vi "AccelerationRetryRoll.vi"(11 "inputInternalData":T5) -> (3 "outputInternalData":T5)   [LabVIEW 2020]
uses:
  Control/AccelerationCurrentRecordIndicator.ctl
  Control/AccelerationBestRecordIndicator.ctl
  CommonControl/Flag.ctl
  Control/AccelerationState.ctl
panel:
  # "Time :"
  # "Entry :"
  # "#1"
  # "#2"
  # "#3"
  # "#4"
  # "Univ. :"
  # "Time :"
  # "Entry :"
  # "#1"
  # "#2"
  # "#3"
  # "#4"
  # "Univ. :"
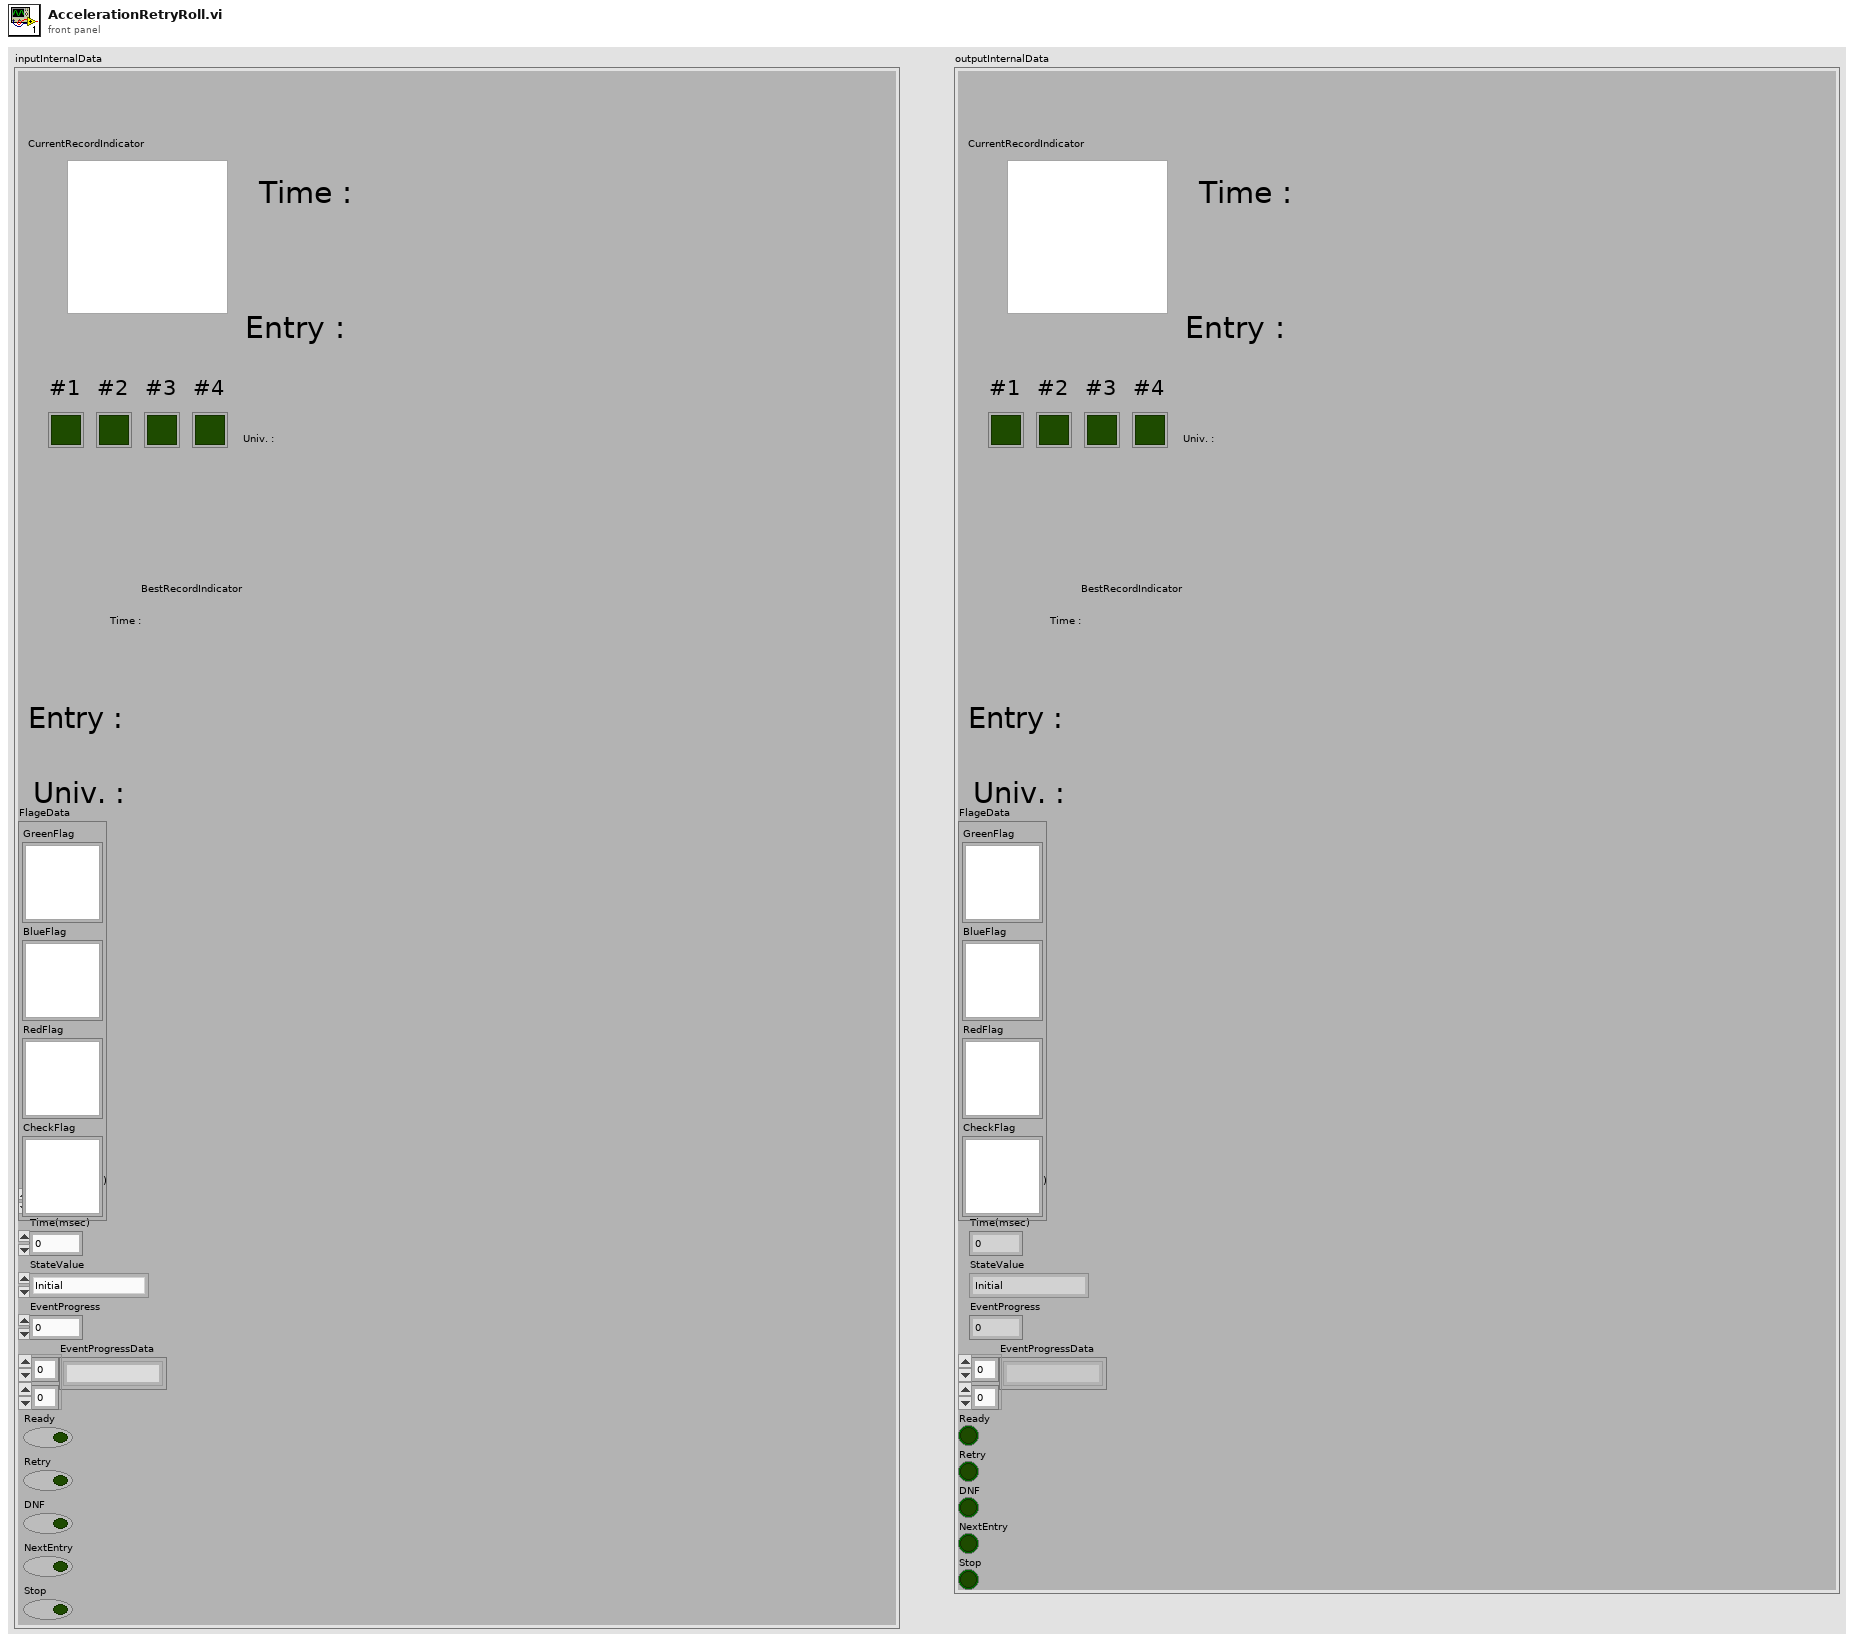
[diagram p1: front panel]
types:
  T1 = typedef "AccelerationCurrentRecordIndicator.ctl" = cluster{"Flag":picture, "Message":string, "Attempt":cluster{"Attempt-1":bool, "Attempt-2":bool, "Attempt-3":bool, "Attempt-4":bool}, "CurrentTime":string, "CurrentEntry":string, "CurrentUniversity":string}
  T2 = typedef "AccelerationBestRecordIndicator.ctl" = cluster{"BestTime":string, "BestEntry":string, "BestUniv":string}
  T3 = typedef "Flag.ctl" = cluster{"GreenFlag":picture, "BlueFlag":picture, "RedFlag":picture, "CheckFlag":picture}
  T4 = typedef "AccelerationState.ctl" = enum16{"Initial", "InputInfomation", "Ready", "Running", "FinshRunning", "LogRecord", "HardwareRelease", "WaittingforNext", "ProgramStop"}
  T5 = cluster{"CurrentRecordIndicator":T1, "BestRecordIndicator":T2, "FlageData":T3, "RefTime(msec)":i64, "Time(msec)":i64, "StateValue":T4, "EventProgress":sgl, "EventProgressData":string[][], "Ready":bool, "Retry":bool, "DNF":bool, "NextEntry":bool, "Stop":bool}
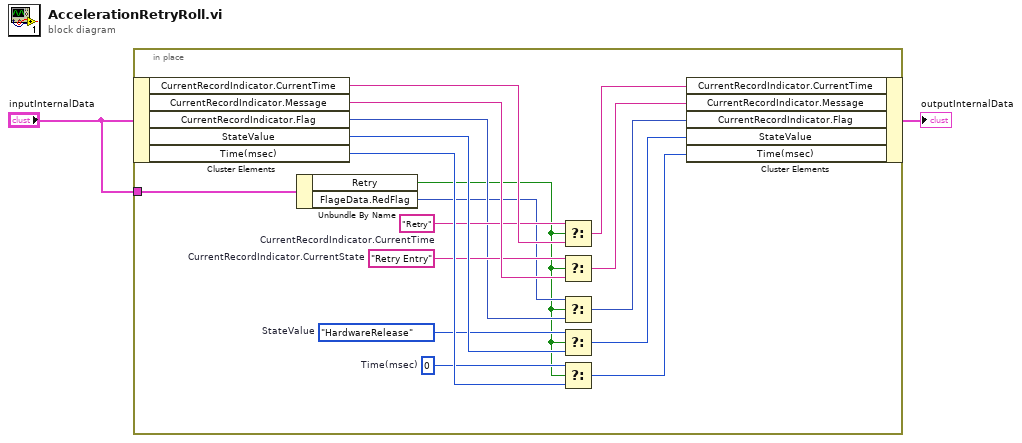
[diagram p0: block diagram]
diagram:
  n1 = in-place {
    in-place-border: "inputInternalData" -> [w19]
    w7 = i64 0  # Time(msec)
    w8 = AccelerationState."HardwareRelease"  # StateValue
    w9 = "Retry Entry"  # CurrentRecordIndicator.CurrentState
    w10 = "Retry"  # CurrentRecordIndicator.CurrentTime
    n2 = in-place-cluster #1("inputInternalData") -> ("CurrentRecordIndicator.CurrentTime"=w18:string, "CurrentRecordIndicator.Message"=w16:string, "CurrentRecordIndicator.Flag"=w6:picture, "StateValue"=w14:T4, "Time(msec)"=w12:i64)
    n3 = Unbundle By Name(w19) -> ("Retry"=w3:bool, "FlageData.RedFlag"=w4:picture)
    n4 = Select(t=w10, s=w3, f=w18) -> (s? t:f=w17:string)
    n5 = Select(t=w9, s=w3, f=w16) -> (s? t:f=w15:string)
    n6 = Select(t=w4, s=w3, f=w6) -> (s? t:f=w5:picture)
    n7 = Select(t=w8, s=w3, f=w14) -> (s? t:f=w13:T4)
    n8 = Select(t=w7, s=w3, f=w12) -> (s? t:f=w11:i64)
    n9 = in-place-cluster #1("CurrentRecordIndicator.CurrentTime"=w17, "CurrentRecordIndicator.Message"=w15, "CurrentRecordIndicator.Flag"=w5, "StateValue"=w13, "Time(msec)"=w11) -> (→"outputInternalData":T5)
  }
